vi "Filter_data_and_calc_speed_171213.vi"(11 "Input array (clean)":dbl[][](array[numeric])) -> (3 "Output":dbl[][](array[numeric]))   [LabVIEW 2018]
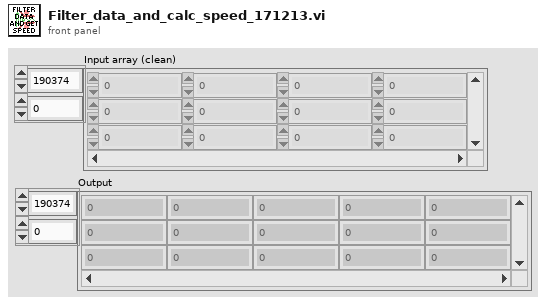
[diagram p1: front panel]
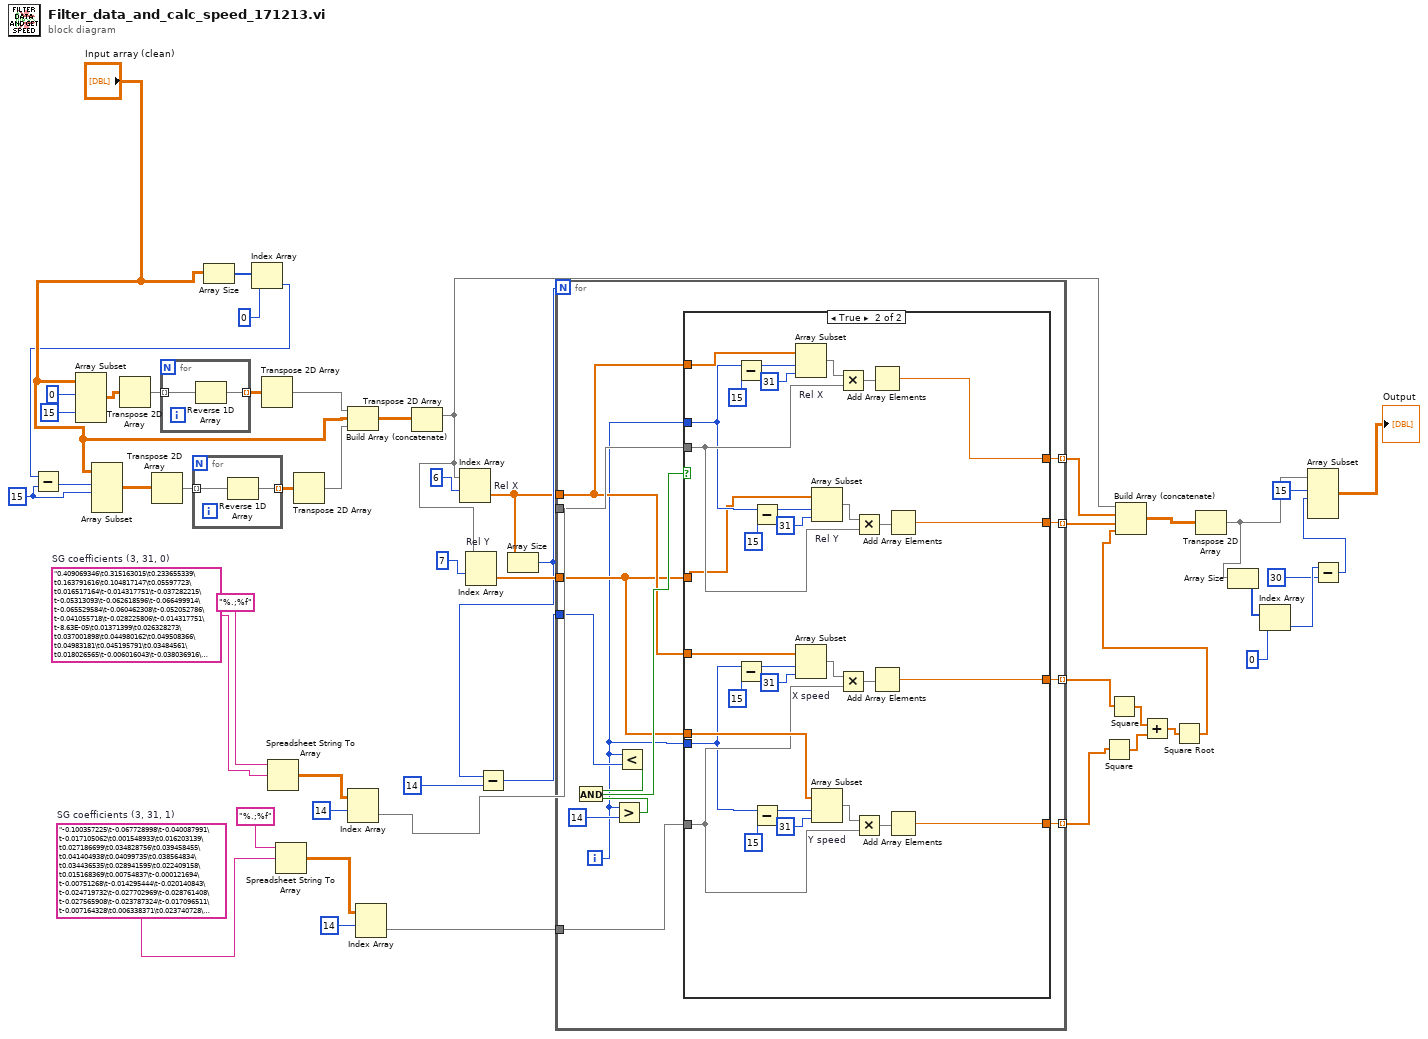
[diagram p0: block diagram]
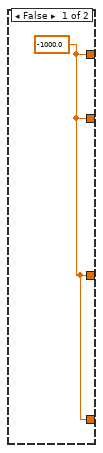
[diagram p2: hidden frame]
diagram:
  w45 = "-0.100357225\t-0.067728998\t-0.040087991\t-0.017105062\t0.001548933\t0.016203139\t0.027186699\t0.034828756\t0.039458455\t0.041404938\t0.04099735\t0.038564834\t0.034436535\t0.028941595\t0.022409158\t0.015168369\t0.00754837\t-0.000121694\t-0.00751268\t-0.014295444\t-0.020140843\t-0.024719732\t-0.027702969\t-0.028761408\t-0.027565908\t-0.023787324\t-0.017096511\t-0.007164328\t0.006338371\t0.023740728\t0.045371888\n-0.08758122\t-0.059696826\t-0.036019671\t-0.01627452\t-0.000186135\t0.01252072\t0.022121282\t0.028890786\t0.033104469\t0.035037569\t0.034965321\t0.033162962\t0.029905728\t0.025468856\t0.020127583\t0.014157144\t0.007832777\t0.001429718\t-0.004776797\t-0.010511531\t-0.015499248\t-0.01946471\t-0.022132683\t-0.023227928\t-0.02247521\t-0.019599292\t-0.014324938\t-0.006376911\t0.004520025\t0.018641107\t0.036261572\n-0.075559916\t-0.052117475\t-0.03215434\t-0.015445464\t-0.001765801\t0.009109696\t0.017406075\t0.023348383\t0.027161666\t0.029070972\t0.029301348\t0.028077841\t0.025625497\t0.022169364\t0.01793449\t0.01314592\t0.008028702\t0.002807883\t-0.002291489\t-0.007044369\t-0.011225708\t-0.01461046\t-0.016973578\t-0.018090015\t-0.017734723\t-0.015682656\t-0.011708766\t-0.005588007\t0.002904668\t0.013994307\t0.027905957\n-0.064293313\t-0.044990944\t-0.028491996\t-0.014617896\t-0.003190067\t0.005970067\t0.01304108\t0.018201547\t0.021630044\t0.023505147\t0.024005431\t0.02330947\t0.021595841\t0.019043119\t0.015829878\t0.012134695\t0.008136145\t0.004012802\t-5.68E-05\t-0.003893958\t-0.007320225\t-0.010156983\t-0.012225656\t-0.013347669\t-0.013344447\t-0.012037414\t-0.009247996\t-0.004797616\t0.0014923\t0.009800328\t0.020305043\n-0.05378141\t-0.038317233\t-0.025032642\t-0.013791815\t-0.00445893\t0.003101832\t0.009026295\t0.013450278\t0.016509605\t0.018340095\t0.01907757\t0.018857852\t0.017816761\t0.01609012\t0.013813749\t0.011123471\t0.008155105\t0.005044474\t0.001927399\t-0.001060299\t-0.003782798\t-0.006104277\t-0.007888915\t-0.00900089\t-0.009304382\t-0.008663568\t-0.006942627\t-0.004005738\t0.00028292\t0.006059169\t0.013458829\n-0.044024208\t-0.032096343\t-0.021776275\t-0.01296722\t-0.005572393\t0.000504993\t0.005361721\t0.009094577\t0.011800347\t0.013575814\t0.014517765\t0.014722984\t0.014288257\t0.013310368\t0.011886102\t0.010112246\t0.008085583\t0.0059029\t0.00366098\t0.00145661\t-0.000613427\t-0.002452344\t-0.003963356\t-0.005049679\t-0.005614527\t-0.005561116\t-0.004792659\t-0.003212373\t-0.000723472\t0.00277083\t0.007367316\n-0.035021707\t-0.026328273\t-0.018722898\t-0.012144113\t-0.006530454\t-0.001820452\t0.002047358\t0.005134443\t0.00750227\t0.009212306\t0.010326016\t0.010904868\t0.011010327\t0.010703862\t0.010046938\t0.009101021\t0.007927579\t0.006588079\t0.005143985\t0.003656767\t0.002187889\t0.000798818\t-0.000448979\t-0.001494035\t-0.002274884\t-0.002730059\t-0.002798093\t-0.002417521\t-0.001526875\t-6.47E-05\t0.002030504\n-0.026773906\t-0.021013024\t-0.015872508\t-0.011322493\t-0.007333113\t-0.003874502\t-0.000916794\t0.001569877\t0.003615376\t0.005249569\t0.006502323\t0.007403502\t0.007982974\t0.008270603\t0.008296255\t0.008089797\t0.007681093\t0.007100011\t0.006376415\t0.005540172\t0.004621148\t0.003649207\t0.002654217\t0.001666042\t0.000714549\t-0.000170396\t-0.000958928\t-0.001621181\t-0.002127289\t-0.002447387\t-0.002551607\n-0.019280806\t-0.016150595\t-0.013225108\t-0.010502361\t-0.007980371\t-0.005657157\t-0.003530735\t-0.001599123\t0.000139663\t0.001687605\t0.003046686\t0.004218888\t0.005206196\t0.00601059\t0.006634055\t0.007078572\t0.007346125\t0.007438697\t0.00735827\t0.007106827\t0.006686351\t0.006098824\t0.00534623\t0.004430552\t0.003353771\t0.002117871\t0.000724835\t-0.000823355\t-0.002524716\t-0.004377264\t-0.006379018\n-0.012542407\t-0.011740987\t-0.010780695\t-0.009683715\t-0.008472228\t-0.007168417\t-0.005794466\t-0.004372555\t-0.002924868\t-0.001473587\t-4.09E-05\t0.001351026\t0.002679993\t0.003923824\t0.005060336\t0.006067348\t0.006922675\t0.007604136\t0.008089549\t0.00835673\t0.008383498\t0.00814767\t0.007627062\t0.006799494\t0.005642782\t0.004134744\t0.002253197\t-2.40E-05\t-0.002719153\t-0.005854321\t-0.009451728\n-0.006558709\t-0.007784199\t-0.008539271\t-0.008866556\t-0.008808683\t-0.008408283\t-0.007707985\t-0.00675042\t-0.005578217\t-0.004234007\t-0.00276042\t-0.001200086\t0.000404366\t0.002010305\t0.0035751\t0.005056123\t0.006410743\t0.007596329\t0.008570252\t0.009289882\t0.009712589\t0.009795743\t0.009496713\t0.008772869\t0.007581582\t0.005880221\t0.003626157\t0.000776759\t-0.002710602\t-0.006878558\t-0.011769737\n-0.001329711\t-0.004280231\t-0.006500836\t-0.008050884\t-0.008989737\t-0.009376754\t-0.009271294\t-0.008732717\t-0.007820385\t-0.006593655\t-0.005111889\t-0.003434446\t-0.001620686\t0.000270032\t0.002178346\t0.004044898\t0.005810328\t0.007415275\t0.00880038\t0.009906283\t0.010673624\t0.011043043\t0.010955181\t0.010350677\t0.009170171\t0.007354304\t0.004843716\t0.001579047\t-0.002499063\t-0.007449974\t-0.013333046\n0.003144586\t-0.001229084\t-0.004665389\t-0.0072367\t-0.009015389\t-0.010073829\t-0.010484391\t-0.010319448\t-0.00965137\t-0.008552531\t-0.007095302\t-0.005352055\t-0.003395162\t-0.001296995\t0.000870074\t0.003033674\t0.005121431\t0.007060975\t0.008779933\t0.010205933\t0.011266603\t0.011889572\t0.012002468\t0.011532917\t0.01040855\t0.008556992\t0.005905874\t0.002382822\t-0.002084535\t-0.00756857\t-0.014141654\n0.006864183\t0.001369243\t-0.00303293\t-0.006424003\t-0.00888564\t-0.01049951\t-0.011347278\t-0.011510611\t-0.011071174\t-0.010110635\t-0.008710659\t-0.006952913\t-0.004919062\t-0.002690774\t-0.000349715\t0.002022449\t0.004344052\t0.006533428\t0.00850891\t0.010188831\t0.011491527\t0.012335329\t0.012638572\t0.012319591\t0.011296717\t0.009488286\t0.00681263\t0.003188084\t-0.001467019\t-0.007234345\t-0.014195561\n0.009829078\t0.003514749\t-0.00160346\t-0.005612792\t-0.00860049\t-0.010653796\t-0.011859954\t-0.012306207\t-0.012079797\t-0.011267967\t-0.00995796\t-0.008237019\t-0.006192387\t-0.003911308\t-0.001481023\t0.001011225\t0.003478191\t0.005832634\t0.007987311\t0.009854978\t0.011348394\t0.012380314\t0.012863496\t0.012710697\t0.011834674\t0.010148184\t0.007563985\t0.003994833\t-0.000646515\t-0.0064473\t-0.013494767\n0.012039273\t0.005207435\t-0.000376979\t-0.004803069\t-0.008159938\t-0.010536688\t-0.012022419\t-0.012706235\t-0.012677237\t-0.012024526\t-0.010837205\t-0.009204374\t-0.007215137\t-0.004958594\t-0.002523848\t-8.23E-19\t0.002523848\t0.004958594\t0.007215137\t0.009204374\t0.010837205\t0.012024526\t0.012677237\t0.012706235\t0.012022419\t0.010536688\t0.008159938\t0.004803069\t0.000376979\t-0.005207435\t-0.012039273\n0.013494767\t0.0064473\t0.000646515\t-0.003994833\t-0.007563985\t-0.010148184\t-0.011834674\t-0.012710697\t-0.012863496\t-0.012380314\t-0.011348394\t-0.009854978\t-0.007987311\t-0.005832634\t-0.003478191\t-0.001011225\t0.001481023\t0.003911308\t0.006192387\t0.008237019\t0.00995796\t0.011267967\t0.012079797\t0.012306207\t0.011859954\t0.010653796\t0.00860049\t0.005612792\t0.00160346\t-0.003514749\t-0.009829078\n0.014195561\t0.007234345\t0.001467019\t-0.003188084\t-0.00681263\t-0.009488286\t-0.011296717\t-0.012319591\t-0.012638572\t-0.012335329\t-0.011491527\t-0.010188831\t-0.00850891\t-0.006533428\t-0.004344052\t-0.002022449\t0.000349715\t0.002690774\t0.004919062\t0.006952913\t0.008710659\t0.010110635\t0.011071174\t0.011510611\t0.011347278\t0.01049951\t0.00888564\t0.006424003\t0.00303293\t-0.001369243\t-0.006864183\n0.014141654\t0.00756857\t0.002084535\t-0.002382822\t-0.005905874\t-0.008556992\t-0.01040855\t-0.011532917\t-0.012002468\t-0.011889572\t-0.011266603\t-0.010205933\t-0.008779933\t-0.007060975\t-0.005121431\t-0.003033674\t-0.000870074\t0.001296995\t0.003395162\t0.005352055\t0.007095302\t0.008552531\t0.00965137\t0.010319448\t0.010484391\t0.010073829\t0.009015389\t0.0072367\t0.004665389\t0.001229084\t-0.003144586\n0.013333046\t0.007449974\t0.002499063\t-0.001579047\t-0.004843716\t-0.007354304\t-0.009170171\t-0.010350677\t-0.010955181\t-0.011043043\t-0.010673624\t-0.009906283\t-0.00880038\t-0.007415275\t-0.005810328\t-0.004044898\t-0.002178346\t-0.000270032\t0.001620686\t0.003434446\t0.005111889\t0.006593655\t0.007820385\t0.008732717\t0.009271294\t0.009376754\t0.008989737\t0.008050884\t0.006500836\t0.004280231\t0.001329711\n0.011769737\t0.006878558\t0.002710602\t-0.000776759\t-0.003626157\t-0.005880221\t-0.007581582\t-0.008772869\t-0.009496713\t-0.009795743\t-0.009712589\t-0.009289882\t-0.008570252\t-0.007596329\t-0.006410743\t-0.005056123\t-0.0035751\t-0.002010305\t-0.000404366\t0.001200086\t0.00276042\t0.004234007\t0.005578217\t0.00675042\t0.007707985\t0.008408283\t0.008808683\t0.008866556\t0.008539271\t0.007784199\t0.006558709\n0.009451728\t0.005854321\t0.002719153\t2.40E-05\t-0.002253197\t-0.004134744\t-0.005642782\t-0.006799494\t-0.007627062\t-0.00814767\t-0.008383498\t-0.00835673\t-0.008089549\t-0.007604136\t-0.006922675\t-0.006067348\t-0.005060336\t-0.003923824\t-0.002679993\t-0.001351026\t4.09E-05\t0.001473587\t0.002924868\t0.004372555\t0.005794466\t0.007168417\t0.008472228\t0.009683715\t0.010780695\t0.011740987\t0.012542407\n0.006379018\t0.004377264\t0.002524716\t0.000823355\t-0.000724835\t-0.002117871\t-0.003353771\t-0.004430552\t-0.00534623\t-0.006098824\t-0.006686351\t-0.007106827\t-0.00735827\t-0.007438697\t-0.007346125\t-0.007078572\t-0.006634055\t-0.00601059\t-0.005206196\t-0.004218888\t-0.003046686\t-0.001687605\t-0.000139663\t0.001599123\t0.003530735\t0.005657157\t0.007980371\t0.010502361\t0.013225108\t0.016150595\t0.019280806\n0.002551607\t0.002447387\t0.002127289\t0.001621181\t0.000958928\t0.000170396\t-0.000714549\t-0.001666042\t-0.002654217\t-0.003649207\t-0.004621148\t-0.005540172\t-0.006376415\t-0.007100011\t-0.007681093\t-0.008089797\t-0.008296255\t-0.008270603\t-0.007982974\t-0.007403502\t-0.006502323\t-0.005249569\t-0.003615376\t-0.001569877\t0.000916794\t0.003874502\t0.007333113\t0.011322493\t0.015872508\t0.021013024\t0.026773906\n-0.002030504\t6.47E-05\t0.001526875\t0.002417521\t0.002798093\t0.002730059\t0.002274884\t0.001494035\t0.000448979\t-0.000798818\t-0.002187889\t-0.003656767\t-0.005143985\t-0.006588079\t-0.007927579\t-0.009101021\t-0.010046938\t-0.010703862\t-0.011010327\t-0.010904868\t-0.010326016\t-0.009212306\t-0.00750227\t-0.005134443\t-0.002047358\t0.001820452\t0.006530454\t0.012144113\t0.018722898\t0.026328273\t0.035021707\n-0.007367316\t-0.00277083\t0.000723472\t0.003212373\t0.004792659\t0.005561116\t0.005614527\t0.005049679\t0.003963356\t0.002452344\t0.000613427\t-0.00145661\t-0.00366098\t-0.0059029\t-0.008085583\t-0.010112246\t-0.011886102\t-0.013310368\t-0.014288257\t-0.014722984\t-0.014517765\t-0.013575814\t-0.011800347\t-0.009094577\t-0.005361721\t-0.000504993\t0.005572393\t0.01296722\t0.021776275\t0.032096343\t0.044024208\n-0.013458829\t-0.006059169\t-0.00028292\t0.004005738\t0.006942627\t0.008663568\t0.009304382\t0.00900089\t0.007888915\t0.006104277\t0.003782798\t0.001060299\t-0.001927399\t-0.005044474\t-0.008155105\t-0.011123471\t-0.013813749\t-0.01609012\t-0.017816761\t-0.018857852\t-0.01907757\t-0.018340095\t-0.016509605\t-0.013450278\t-0.009026295\t-0.003101832\t0.00445893\t0.013791815\t0.025032642\t0.038317233\t0.05378141\n-0.020305043\t-0.009800328\t-0.0014923\t0.004797616\t0.009247996\t0.012037414\t0.013344447\t0.013347669\t0.012225656\t0.010156983\t0.007320225\t0.003893958\t5.68E-05\t-0.004012802\t-0.008136145\t-0.012134695\t-0.015829878\t-0.019043119\t-0.021595841\t-0.02330947\t-0.024005431\t-0.023505147\t-0.021630044\t-0.018201547\t-0.01304108\t-0.005970067\t0.003190067\t0.014617896\t0.028491996\t0.044990944\t0.064293313\n-0.027905957\t-0.013994307\t-0.002904668\t0.005588007\t0.011708766\t0.015682656\t0.017734723\t0.018090015\t0.016973578\t0.01461046\t0.011225708\t0.007044369\t0.002291489\t-0.002807883\t-0.008028702\t-0.01314592\t-0.01793449\t-0.022169364\t-0.025625497\t-0.028077841\t-0.029301348\t-0.029070972\t-0.027161666\t-0.023348383\t-0.017406075\t-0.009109696\t0.001765801\t0.015445464\t0.03215434\t0.052117475\t0.075559916\n-0.036261572\t-0.018641107\t-0.004520025\t0.006376911\t0.014324938\t0.019599292\t0.02247521\t0.023227928\t0.022132683\t0.01946471\t0.015499248\t0.010511531\t0.004776797\t-0.001429718\t-0.007832777\t-0.014157144\t-0.020127583\t-0.025468856\t-0.029905728\t-0.033162962\t-0.034965321\t-0.035037569\t-0.033104469\t-0.028890786\t-0.022121282\t-0.01252072\t0.000186135\t0.01627452\t0.036019671\t0.059696826\t0.08758122\n-0.045371888\t-0.023740728\t-0.006338371\t0.007164328\t0.017096511\t0.023787324\t0.027565908\t0.028761408\t0.027702969\t0.024719732\t0.020140843\t0.014295444\t0.00751268\t0.000121694\t-0.00754837\t-0.015168369\t-0.022409158\t-0.028941595\t-0.034436535\t-0.038564834\t-0.04099735\t-0.041404938\t-0.039458455\t-0.034828756\t-0.027186699\t-0.016203139\t-0.001548933\t0.017105062\t0.040087991\t0.067728998\t0.100357225"  # SG coefficients (3, 31, 1)
  w20 = 15 ("length")
  w41 = "0.409069346\t0.315163015\t0.233655339\t0.163791616\t0.104817147\t0.05597723\t0.016517164\t-0.014317751\t-0.037282215\t-0.05313093\t-0.062618596\t-0.066499914\t-0.065529584\t-0.060462308\t-0.052052786\t-0.041055718\t-0.028225806\t-0.014317751\t-8.63E-05\t0.01371399\t0.026328273\t0.037001898\t0.044980162\t0.049508366\t0.04983181\t0.045195791\t0.03484561\t0.018026565\t-0.006016043\t-0.038036916\t-0.078790754\n0.315163015\t0.251487839\t0.195618423\t0.147101949\t0.105485596\t0.070316543\t0.04114197\t0.017509056\t-0.001035018\t-0.014943074\t-0.024667932\t-0.030662412\t-0.033379334\t-0.03327152\t-0.030791789\t-0.026392962\t-0.020527859\t-0.013649301\t-0.006210109\t0.001336898\t0.008538899\t0.014943074\t0.020096602\t0.023546662\t0.024840435\t0.023525099\t0.019147835\t0.011255822\t-0.000603761\t-0.016883733\t-0.038036916\n0.233655339\t0.195618423\t0.161548334\t0.131242081\t0.104496678\t0.081109135\t0.060876464\t0.043595677\t0.029063784\t0.017077799\t0.007434731\t-6.84E-05\t-0.005634603\t-0.009466847\t-0.011768126\t-0.01274143\t-0.012589746\t-0.011516064\t-0.009723371\t-0.007414656\t-0.004792907\t-0.002061114\t0.000577736\t0.002920655\t0.004764652\t0.005906741\t0.006143933\t0.005273239\t0.00309167\t-0.000603761\t-0.006016043\n0.163791616\t0.147101949\t0.131242081\t0.116210525\t0.102005794\t0.0886264\t0.076070857\t0.064337678\t0.053425375\t0.043332461\t0.034057449\t0.025598853\t0.017955185\t0.011124958\t0.005106684\t-0.000101122\t-0.004499949\t-0.008091284\t-0.010876613\t-0.012857423\t-0.014035203\t-0.014411438\t-0.013987615\t-0.012765223\t-0.010745748\t-0.007930678\t-0.004321498\t8.03E-05\t0.005273239\t0.011255822\t0.018026565\n0.104817147\t0.105485596\t0.104496678\t0.102005794\t0.098168345\t0.093139733\t0.08707536\t0.080130626\t0.072460934\t0.064221684\t0.055568278\t0.046656118\t0.037640605\t0.02867714\t0.019921124\t0.01152796\t0.003653049\t-0.003548209\t-0.009920411\t-0.015308156\t-0.019556043\t-0.02250867\t-0.024010636\t-0.023906539\t-0.022040978\t-0.018258552\t-0.012403859\t-0.004321498\t0.006143933\t0.019147835\t0.03484561\n0.05597723\t0.070316543\t0.081109135\t0.0886264\t0.093139733\t0.09492053\t0.094240184\t0.09137009\t0.086581644\t0.080146241\t0.072335274\t0.06342014\t0.053672232\t0.043362946\t0.032763677\t0.022145819\t0.011780767\t0.001939915\t-0.00710534\t-0.015083604\t-0.021723484\t-0.026753582\t-0.029902506\t-0.03089886\t-0.029471249\t-0.025348278\t-0.018258552\t-0.007930678\t0.005906741\t0.023525099\t0.045195791\n0.016517164\t0.04114197\t0.060876464\t0.076070857\t0.08707536\t0.094240184\t0.097915539\t0.098451637\t0.096198688\t0.091506903\t0.084726493\t0.07620767\t0.066300643\t0.055355624\t0.043722823\t0.031752452\t0.019794721\t0.008199842\t-0.002681976\t-0.01250052\t-0.020905581\t-0.027546948\t-0.032074408\t-0.034137753\t-0.03338677\t-0.029471249\t-0.022040978\t-0.010745748\t0.004764652\t0.024840435\t0.04983181\n-0.014317751\t0.017509056\t0.043595677\t0.064337678\t0.080130626\t0.09137009\t0.098451637\t0.101770833\t0.101723246\t0.098704443\t0.093109991\t0.085335459\t0.075776412\t0.064828419\t0.052887046\t0.040347861\t0.027606431\t0.015058324\t0.003099106\t-0.007875655\t-0.017470392\t-0.025289537\t-0.030937524\t-0.034018785\t-0.034137753\t-0.03089886\t-0.023906539\t-0.012765223\t0.002920655\t0.023546662\t0.049508366\n-0.037282215\t-0.001035018\t0.029063784\t0.053425375\t0.072460934\t0.086581644\t0.096198688\t0.101723246\t0.1035665\t0.102139632\t0.097853825\t0.091120258\t0.082350116\t0.071954578\t0.060344828\t0.047932046\t0.035127414\t0.022342115\t0.00998733\t-0.001525759\t-0.011785971\t-0.020382124\t-0.026903035\t-0.030937524\t-0.032074408\t-0.029902506\t-0.024010636\t-0.013987615\t0.000577736\t0.020096602\t0.044980162\n-0.05313093\t-0.014943074\t0.017077799\t0.043332461\t0.064221684\t0.080146241\t0.091506903\t0.098704443\t0.102139632\t0.102213243\t0.099326049\t0.09387882\t0.086272329\t0.076907348\t0.06618465\t0.054505006\t0.042269188\t0.029877969\t0.017732121\t0.006232415\t-0.004220376\t-0.013225479\t-0.020382124\t-0.025289537\t-0.027546948\t-0.026753582\t-0.02250867\t-0.014411438\t-0.002061114\t0.014943074\t0.037001898\n-0.062618596\t-0.024667932\t0.007434731\t0.034057449\t0.055568278\t0.072335274\t0.084726493\t0.093109991\t0.097853825\t0.099326049\t0.09789472\t0.093927894\t0.087793627\t0.079859975\t0.070494994\t0.060066741\t0.04894327\t0.037492639\t0.026082903\t0.015082117\t0.004858339\t-0.004220376\t-0.011785971\t-0.017470392\t-0.020905581\t-0.021723484\t-0.019556043\t-0.014035203\t-0.004792907\t0.008538899\t0.026328273\n-0.066499914\t-0.030662412\t-6.84E-05\t0.025598853\t0.046656118\t0.06342014\t0.07620767\t0.085335459\t0.091120258\t0.09387882\t0.093927894\t0.091584232\t0.087164586\t0.080985706\t0.073364344\t0.064617251\t0.055061179\t0.045012878\t0.0347891\t0.024706596\t0.015082117\t0.006232415\t-0.001525759\t-0.007875655\t-0.01250052\t-0.015083604\t-0.015308156\t-0.012857423\t-0.007414656\t0.001336898\t0.01371399\n-0.065529584\t-0.033379334\t-0.005634603\t0.017955185\t0.037640605\t0.053672232\t0.066300643\t0.075776412\t0.082350116\t0.086272329\t0.087793627\t0.087164586\t0.084635781\t0.080457787\t0.074881181\t0.068156538\t0.060534432\t0.052265441\t0.043600138\t0.0347891\t0.026082903\t0.017732121\t0.00998733\t0.003099106\t-0.002681976\t-0.00710534\t-0.009920411\t-0.010876613\t-0.009723371\t-0.006210109\t-8.63E-05\n-0.060462308\t-0.03327152\t-0.009466847\t0.011124958\t0.02867714\t0.043362946\t0.055355624\t0.064828419\t0.071954578\t0.076907348\t0.079859975\t0.080985706\t0.080457787\t0.078449466\t0.075133987\t0.070684599\t0.065274547\t0.059077079\t0.052265441\t0.045012878\t0.037492639\t0.029877969\t0.022342115\t0.015058324\t0.008199842\t0.001939915\t-0.003548209\t-0.008091284\t-0.011516064\t-0.013649301\t-0.014317751\n-0.052052786\t-0.030791789\t-0.011768126\t0.005106684\t0.019921124\t0.032763677\t0.043722823\t0.052887046\t0.060344828\t0.06618465\t0.070494994\t0.073364344\t0.074881181\t0.075133987\t0.074211245\t0.072201436\t0.069193043\t0.065274547\t0.060534432\t0.055061179\t0.04894327\t0.042269188\t0.035127414\t0.027606431\t0.019794721\t0.011780767\t0.003653049\t-0.004499949\t-0.012589746\t-0.020527859\t-0.028225806\n-0.041055718\t-0.026392962\t-0.01274143\t-0.000101122\t0.01152796\t0.022145819\t0.031752452\t0.040347861\t0.047932046\t0.054505006\t0.060066741\t0.064617251\t0.068156538\t0.070684599\t0.072201436\t0.072707048\t0.072201436\t0.070684599\t0.068156538\t0.064617251\t0.060066741\t0.054505006\t0.047932046\t0.040347861\t0.031752452\t0.022145819\t0.01152796\t-0.000101122\t-0.01274143\t-0.026392962\t-0.041055718\n-0.028225806\t-0.020527859\t-0.012589746\t-0.004499949\t0.003653049\t0.011780767\t0.019794721\t0.027606431\t0.035127414\t0.042269188\t0.04894327\t0.055061179\t0.060534432\t0.065274547\t0.069193043\t0.072201436\t0.074211245\t0.075133987\t0.074881181\t0.073364344\t0.070494994\t0.06618465\t0.060344828\t0.052887046\t0.043722823\t0.032763677\t0.019921124\t0.005106684\t-0.011768126\t-0.030791789\t-0.052052786\n-0.014317751\t-0.013649301\t-0.011516064\t-0.008091284\t-0.003548209\t0.001939915\t0.008199842\t0.015058324\t0.022342115\t0.029877969\t0.037492639\t0.045012878\t0.052265441\t0.059077079\t0.065274547\t0.070684599\t0.075133987\t0.078449466\t0.080457787\t0.080985706\t0.079859975\t0.076907348\t0.071954578\t0.064828419\t0.055355624\t0.043362946\t0.02867714\t0.011124958\t-0.009466847\t-0.03327152\t-0.060462308\n-8.63E-05\t-0.006210109\t-0.009723371\t-0.010876613\t-0.009920411\t-0.00710534\t-0.002681976\t0.003099106\t0.00998733\t0.017732121\t0.026082903\t0.0347891\t0.043600138\t0.052265441\t0.060534432\t0.068156538\t0.074881181\t0.080457787\t0.084635781\t0.087164586\t0.087793627\t0.086272329\t0.082350116\t0.075776412\t0.066300643\t0.053672232\t0.037640605\t0.017955185\t-0.005634603\t-0.033379334\t-0.065529584\n0.01371399\t0.001336898\t-0.007414656\t-0.012857423\t-0.015308156\t-0.015083604\t-0.01250052\t-0.007875655\t-0.001525759\t0.006232415\t0.015082117\t0.024706596\t0.0347891\t0.045012878\t0.055061179\t0.064617251\t0.073364344\t0.080985706\t0.087164586\t0.091584232\t0.093927894\t0.09387882\t0.091120258\t0.085335459\t0.07620767\t0.06342014\t0.046656118\t0.025598853\t-6.84E-05\t-0.030662412\t-0.066499914\n0.026328273\t0.008538899\t-0.004792907\t-0.014035203\t-0.019556043\t-0.021723484\t-0.020905581\t-0.017470392\t-0.011785971\t-0.004220376\t0.004858339\t0.015082117\t0.026082903\t0.037492639\t0.04894327\t0.060066741\t0.070494994\t0.079859975\t0.087793627\t0.093927894\t0.09789472\t0.099326049\t0.097853825\t0.093109991\t0.084726493\t0.072335274\t0.055568278\t0.034057449\t0.007434731\t-0.024667932\t-0.062618596\n0.037001898\t0.014943074\t-0.002061114\t-0.014411438\t-0.02250867\t-0.026753582\t-0.027546948\t-0.025289537\t-0.020382124\t-0.013225479\t-0.004220376\t0.006232415\t0.017732121\t0.029877969\t0.042269188\t0.054505006\t0.06618465\t0.076907348\t0.086272329\t0.09387882\t0.099326049\t0.102213243\t0.102139632\t0.098704443\t0.091506903\t0.080146241\t0.064221684\t0.043332461\t0.017077799\t-0.014943074\t-0.05313093\n0.044980162\t0.020096602\t0.000577736\t-0.013987615\t-0.024010636\t-0.029902506\t-0.032074408\t-0.030937524\t-0.026903035\t-0.020382124\t-0.011785971\t-0.001525759\t0.00998733\t0.022342115\t0.035127414\t0.047932046\t0.060344828\t0.071954578\t0.082350116\t0.091120258\t0.097853825\t0.102139632\t0.1035665\t0.101723246\t0.096198688\t0.086581644\t0.072460934\t0.053425375\t0.029063784\t-0.001035018\t-0.037282215\n0.049508366\t0.023546662\t0.002920655\t-0.012765223\t-0.023906539\t-0.03089886\t-0.034137753\t-0.034018785\t-0.030937524\t-0.025289537\t-0.017470392\t-0.007875655\t0.003099106\t0.015058324\t0.027606431\t0.040347861\t0.052887046\t0.064828419\t0.075776412\t0.085335459\t0.093109991\t0.098704443\t0.101723246\t0.101770833\t0.098451637\t0.09137009\t0.080130626\t0.064337678\t0.043595677\t0.017509056\t-0.014317751\n0.04983181\t0.024840435\t0.004764652\t-0.010745748\t-0.022040978\t-0.029471249\t-0.03338677\t-0.034137753\t-0.032074408\t-0.027546948\t-0.020905581\t-0.01250052\t-0.002681976\t0.008199842\t0.019794721\t0.031752452\t0.043722823\t0.055355624\t0.066300643\t0.07620767\t0.084726493\t0.091506903\t0.096198688\t0.098451637\t0.097915539\t0.094240184\t0.08707536\t0.076070857\t0.060876464\t0.04114197\t0.016517164\n0.045195791\t0.023525099\t0.005906741\t-0.007930678\t-0.018258552\t-0.025348278\t-0.029471249\t-0.03089886\t-0.029902506\t-0.026753582\t-0.021723484\t-0.015083604\t-0.00710534\t0.001939915\t0.011780767\t0.022145819\t0.032763677\t0.043362946\t0.053672232\t0.06342014\t0.072335274\t0.080146241\t0.086581644\t0.09137009\t0.094240184\t0.09492053\t0.093139733\t0.0886264\t0.081109135\t0.070316543\t0.05597723\n0.03484561\t0.019147835\t0.006143933\t-0.004321498\t-0.012403859\t-0.018258552\t-0.022040978\t-0.023906539\t-0.024010636\t-0.02250867\t-0.019556043\t-0.015308156\t-0.009920411\t-0.003548209\t0.003653049\t0.01152796\t0.019921124\t0.02867714\t0.037640605\t0.046656118\t0.055568278\t0.064221684\t0.072460934\t0.080130626\t0.08707536\t0.093139733\t0.098168345\t0.102005794\t0.104496678\t0.105485596\t0.104817147\n0.018026565\t0.011255822\t0.005273239\t8.03E-05\t-0.004321498\t-0.007930678\t-0.010745748\t-0.012765223\t-0.013987615\t-0.014411438\t-0.014035203\t-0.012857423\t-0.010876613\t-0.008091284\t-0.004499949\t-0.000101122\t0.005106684\t0.011124958\t0.017955185\t0.025598853\t0.034057449\t0.043332461\t0.053425375\t0.064337678\t0.076070857\t0.0886264\t0.102005794\t0.116210525\t0.131242081\t0.147101949\t0.163791616\n-0.006016043\t-0.000603761\t0.00309167\t0.005273239\t0.006143933\t0.005906741\t0.004764652\t0.002920655\t0.000577736\t-0.002061114\t-0.004792907\t-0.007414656\t-0.009723371\t-0.011516064\t-0.012589746\t-0.01274143\t-0.011768126\t-0.009466847\t-0.005634603\t-6.84E-05\t0.007434731\t0.017077799\t0.029063784\t0.043595677\t0.060876464\t0.081109135\t0.104496678\t0.131242081\t0.161548334\t0.195618423\t0.233655339\n-0.038036916\t-0.016883733\t-0.000603761\t0.011255822\t0.019147835\t0.023525099\t0.024840435\t0.023546662\t0.020096602\t0.014943074\t0.008538899\t0.001336898\t-0.006210109\t-0.013649301\t-0.020527859\t-0.026392962\t-0.030791789\t-0.03327152\t-0.033379334\t-0.030662412\t-0.024667932\t-0.014943074\t-0.001035018\t0.017509056\t0.04114197\t0.070316543\t0.105485596\t0.147101949\t0.195618423\t0.251487839\t0.315163015\n-0.078790754\t-0.038036916\t-0.006016043\t0.018026565\t0.03484561\t0.045195791\t0.04983181\t0.049508366\t0.044980162\t0.037001898\t0.026328273\t0.01371399\t-8.63E-05\t-0.014317751\t-0.028225806\t-0.041055718\t-0.052052786\t-0.060462308\t-0.065529584\t-0.066499914\t-0.062618596\t-0.05313093\t-0.037282215\t-0.014317751\t0.016517164\t0.05597723\t0.104817147\t0.163791616\t0.233655339\t0.315163015\t0.409069346\n"  # SG coefficients (3, 31, 0)
  n1 = Array Subset(array="Input array (clean)", index (row)=0 ("index"), length (row)=15 ("length")) -> (w17:dbl[][])  [unwired: 2 in]
  n2 = Transpose 2D Array(2D array=w17) -> (transposed array=w16:dbl[][])
  n3 = for {
    tunnel: w16 -> [w54] mode=indexing
    tunnel: [w53] -> w15 mode=indexing
    n4 = Reverse 1D Array(array=w54) -> (reversed array=w53:dbl[])
  }
  n5 = Array Size(array="Input array (clean)") -> (size(s)=w11:i32[])
  n6 = Index Array(array=w11, index=0) -> (element=w19:i32)
  n7 = Subtract(x=w19, y=w20) -> (x-y=w18:i32)
  n8 = Array Subset(array="Input array (clean)", index (row)=w18, length (row)=w20) -> (w23:dbl[][])  [unwired: 2 in]
  n9 = Transpose 2D Array(2D array=w23) -> (transposed array=w22:dbl[][])
  n10 = for {
    tunnel: w22 -> [w56] mode=indexing
    tunnel: [w55] -> w21 mode=indexing
    n11 = Reverse 1D Array(array=w56) -> (reversed array=w55:dbl[])
  }
  n12 = Transpose 2D Array(2D array=w15) -> (transposed array=w24:dbl[][])
  n13 = Spreadsheet String To Array(format string="%.;%f", spreadsheet string=w41) -> (array=w33:dbl[][])  [unwired: 2 in]
  n14 = Spreadsheet String To Array(format string="%.;%f", spreadsheet string=w45) -> (array=w44:dbl[][])  [unwired: 2 in]
  n15 = Transpose 2D Array(2D array=w21) -> (transposed array=w25:dbl[][])
  n16 = Build Array (concatenate)(w24, "Input array (clean)", w25) -> (w27:dbl[][])
  n17 = Index Array(array=w33, index (row)=14) -> (element=w34:dbl[])  [unwired: 1 in]
  n18 = Index Array(array=w44, index (row)=14) -> (element=w46:dbl[])  [unwired: 1 in]
  n19 = Transpose 2D Array(2D array=w27) -> (transposed array=w38:dbl[][])
  n20 = Index Array "Rel X"(array=w38, index (row)=6) -> (element=w29:dbl[])  [unwired: 1 in]
  n21 = Index Array "Rel Y"(array=w38, index (row)=7) -> (element=w39:dbl[])  [unwired: 1 in]
  n22 = Array Size(array=w29) -> (size(s)=w35:i32)
  n23 = Subtract(x=w35, y=14) -> (x-y=w31:i32)
  n24 = for {
    N: w35 -> [_]
    tunnel: w29 -> [w62]
    tunnel: w31 -> [w69]
    tunnel: w34 -> [w66]
    tunnel: [w65] -> w36 mode=indexing
    tunnel: w39 -> [w61]
    tunnel: [w64] -> w40 mode=indexing
    tunnel: w46 -> [w60]
    tunnel: [w58] -> w48 mode=indexing
    tunnel: [w57] -> w49 mode=indexing
    i -> [w59]
    n25 = Greater?(x=w59, y=14) -> (0:w63:bool)
    n26 = Less?(x=w59, y=w69) -> (x < y?=w68:bool)
    n27 = And(x=w68, y=w63) -> (x .and. y?=w67:bool)
    n28 = case shown="True" w67 {
      tunnel: w62 -> [_ w103]
      tunnel: w59 -> [_ w90]
      tunnel: w66 -> [_ w91]
      tunnel: [w71 w97] -> w65
      tunnel: w61 -> [_ w89]
      tunnel: [w71 w88] -> w64
      tunnel: w62 -> [_ w77]
      tunnel: w61 -> [_ w76]
      tunnel: w60 -> [_ w75]
      tunnel: w59 -> [_ w74]
      tunnel: [w71 w73] -> w58
      tunnel: [w71 w72] -> w57
      frame False {
        w71 = -1000.0
      }
      frame True {
        n29 = Subtract(x=w90, y=15) -> (x-y=w101:i32)
        n30 = Subtract(x=w74, y=15) -> (x-y=w86:i32)
        n31 = Subtract(x=w90, y=15) -> (x-y=w95:i32)
        n32 = Subtract(x=w74, y=15) -> (x-y=w81:i32)
        n33 = Array Subset "Rel X"(array=w103, index=w101, length=31) -> (w99:dbl[])
        n34 = Array Subset "X speed"(array=w77, index=w86, length=31) -> (w84:dbl[])
        n35 = Array Subset "Rel Y"(array=w89, index=w95, length=31) -> (w93:dbl[])
        n36 = Array Subset "Y speed"(array=w76, index=w81, length=31) -> (w79:dbl[])
        n37 = Multiply(x=w99, y=w91) -> (x*y=w98:dbl[])
        n38 = Multiply(x=w84, y=w75) -> (x*y=w83:dbl[])
        n39 = Multiply(x=w93, y=w91) -> (x*y=w92:dbl[])
        n40 = Multiply(x=w79, y=w75) -> (x*y=w78:dbl[])
        n41 = Add Array Elements(numeric array=w98) -> (sum=w97:dbl)
        n42 = Add Array Elements(numeric array=w83) -> (sum=w73:dbl)
        n43 = Add Array Elements(numeric array=w92) -> (sum=w88:dbl)
        n44 = Add Array Elements(numeric array=w78) -> (sum=w72:dbl)
      }
    }
  }
  n45 = Square(x=w49) -> (x^2=w51:dbl[])
  n46 = Square(x=w48) -> (x^2=w50:dbl[])
  n47 = Add(x=w50, y=w51) -> (x+y=w52:dbl[])
  n48 = Square Root(x=w52) -> (sqrt(x)=w1:dbl[])
  n49 = Build Array (concatenate)(w38, w36, w40, w1) -> (w47:dbl[][])
  n50 = Transpose 2D Array(2D array=w47) -> (transposed array=w7:dbl[][])
  n51 = Array Size(array=w7) -> (size(s)=w6:i32[])
  n52 = Index Array(array=w6, index=0) -> (element=w5:i32)
  n53 = Subtract(x=w5, y=30) -> (x-y=w3:i32)
  n54 = Array Subset(array=w7, index (row)=15 ("index"), length (row)=w3) -> (→"Output":dbl[][])  [unwired: 2 in]
